vi "SLSC Parse Capabilities File.vi"(8 "error in":errorcluster, 11 "module capabilities JSON string":string) -> (0 "error out":errorcluster, 3 "SLSC EDS module":T1)   [LabVIEW 2015]
doc: "This SLSC capabilities string parser deserializes a module's JSON capabilities string as read using SLSC Read NVMEM.vi example (*.bin)) and converts it to a cluster."
uses:
  EDSjsonStructure.ctl
  enum.ctl
  property.ctl
  command.ctl
  scale.ctl
  physicalChannel.ctl
  register.ctl
  <vilib>/addons/_JKI.lib/Serialization/JSON/JKI JSON Serialization.lvlib
panel:
  out "First Region":string
  out "raw?":bool
  out "result string":string
  # "not working\nregisterMap->registers->initialValue"
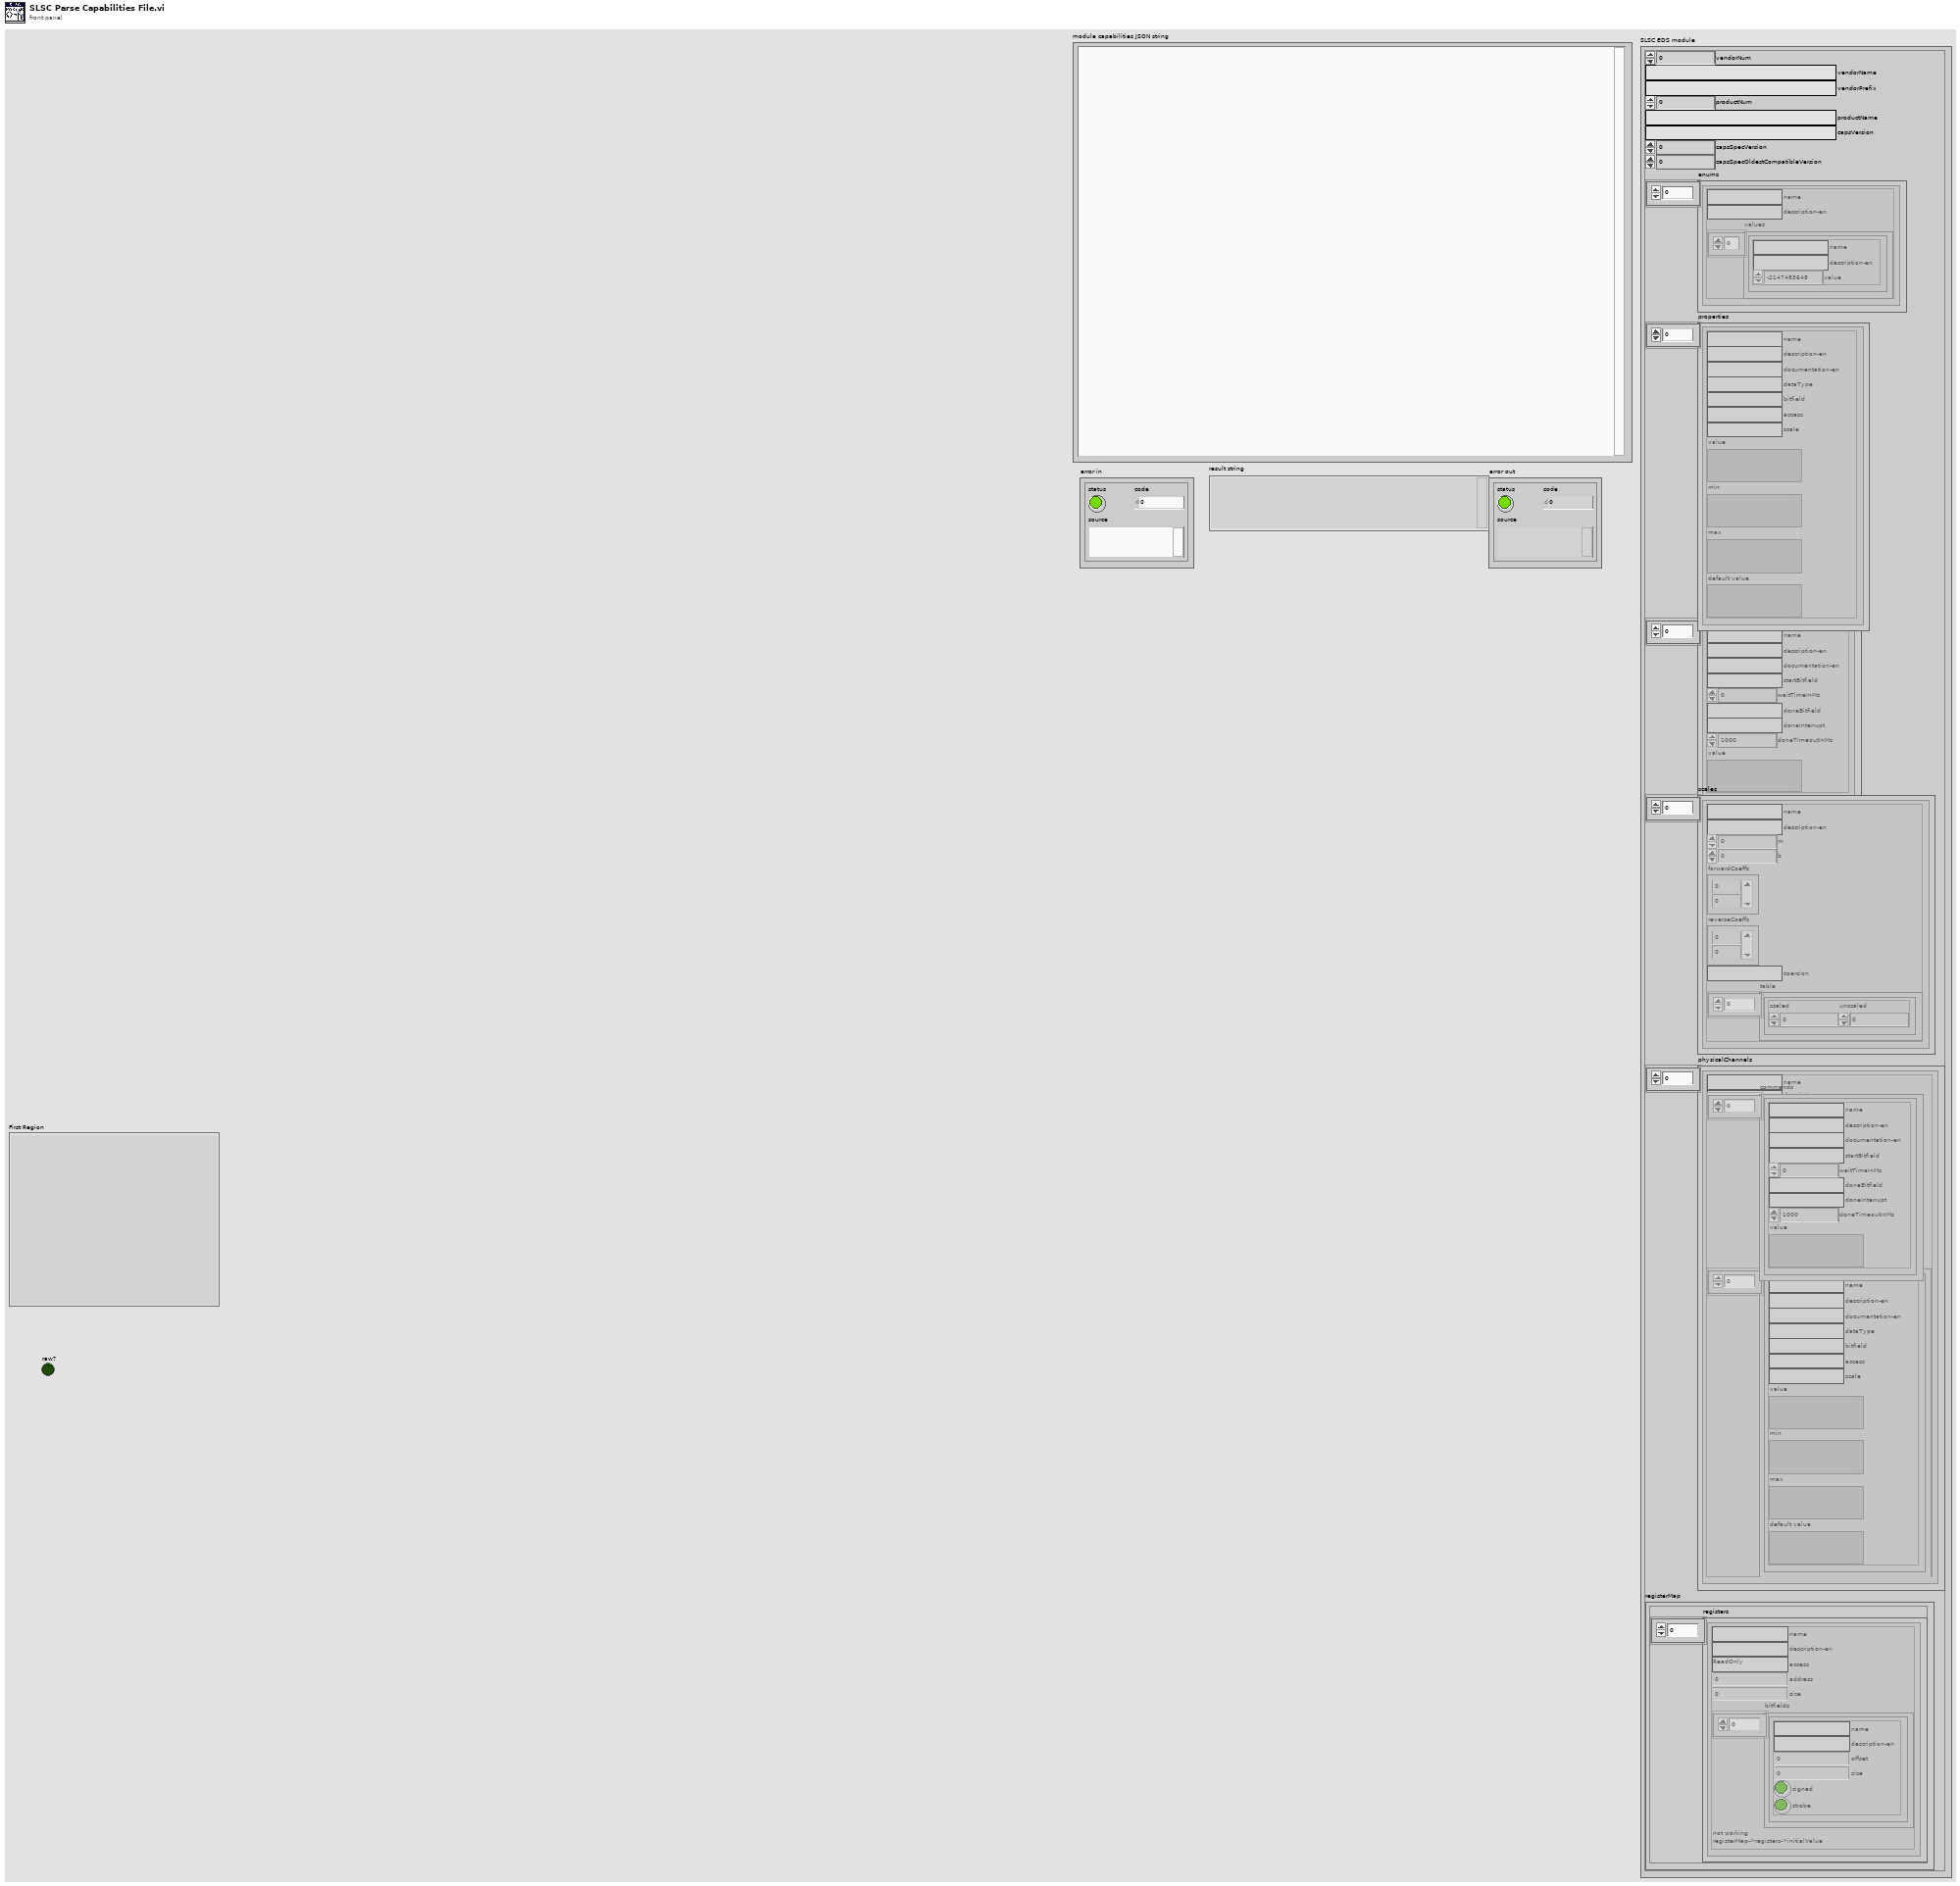
[diagram p1: front panel]
types:
  T1 = typedef "EDSjsonStructure.ctl" = cluster{"vendorNum":u32, "vendorName":string, "vendorPrefix":string, "productNum":u32, "productName":string, "capsVersion":string, "capsSpecVersion":u32, "capsSpecOldestCompatibleVersion":u32, "enums":T2[], "properties":T3[], "commands":T4[], "scales":T5[], "physicalChannels":T6[], "registerMap":cluster{"registers":T7[]}}
  T2 = typedef "enum.ctl" = cluster{"name":string, "description-en":string, "values":cluster{"name":string, "description-en":string, "value":i32}[]}
  T3 = typedef "property.ctl" = cluster{"name":string, "description-en":string, "documentation-en":string, "dataType":string, "bitfield":string, "access":string, "scale":string, "value":variant, "min":variant, "max":variant, "default value":variant}
  T4 = typedef "command.ctl" = cluster{"name":string, "description-en":string, "documentation-en":string, "startBitfield":string, "waitTimeInMs":i32, "doneBitfield":string, "doneInterrupt":string, "doneTimeoutInMs":i32, "value":variant}
  T5 = typedef "scale.ctl" = cluster{"name":string, "description-en":string, "m":dbl, "b":dbl, "forwardCoeffs":dbl[], "reverseCoeffs":dbl[], "coercion":string, "table":cluster{"scaled":dbl, "unscaled":dbl}[]}
  T6 = typedef "physicalChannel.ctl" = cluster{"name":string, "description-en":string, "commands":T4[], "properties":T3[]}
  T7 = typedef "register.ctl" = cluster{"name":string, "description-en":string, "access":string, "address":u32, "size":u32, "bitfields":cluster{"name":string, "description-en":string, "offset":u32, "size":u32, "signed":bool, "strobe":bool}[]}
  T8 = cluster{"areas":cluster{"name":string, "offsets":i32[], "size":i32}[]}
  T9 = cluster{"name":string, "offsets":i32[], "size":i32}[]
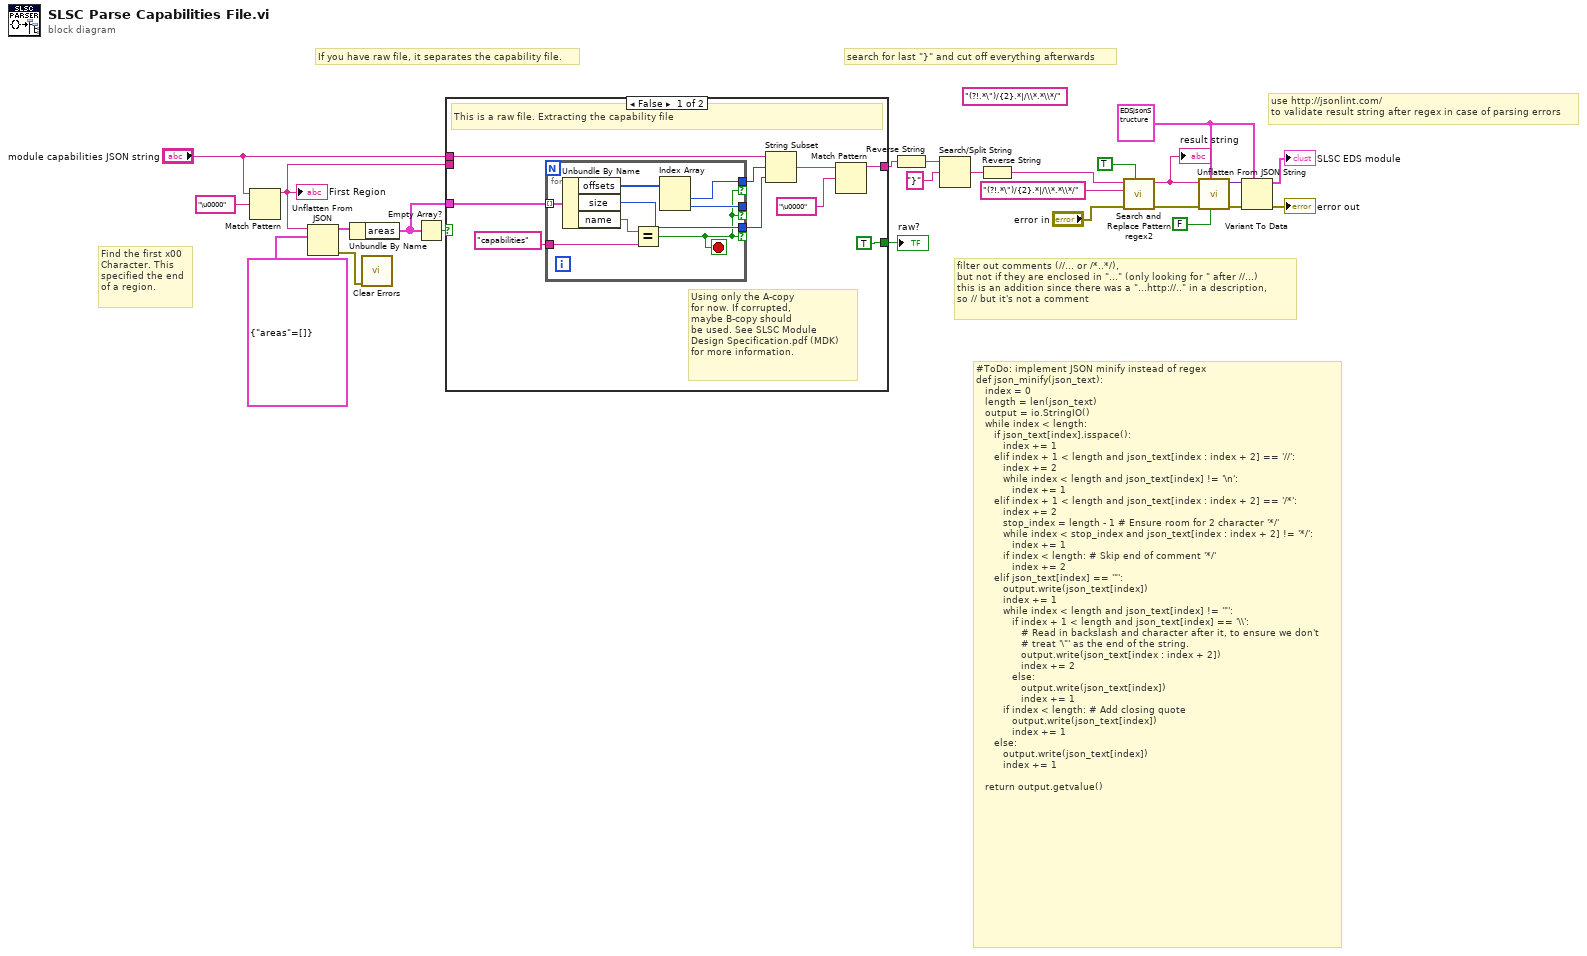
[diagram p0: block diagram]
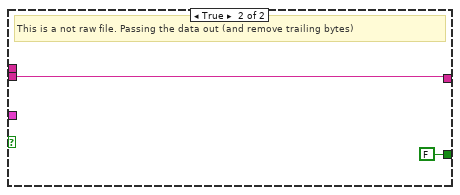
[diagram p2: hidden frame]
diagram:
  (unwired) "(?!.*\")/{2}.*|/\\*.*\\*/" ("regular expression (\"\")")
  w19 = T1 {"vendorNum"=0, "vendorName"="", "vendorPrefix"="", "productNum"=0, "productName"="", "capsVersion"="", "capsSpecVersion"=0, "capsSpecOldestCompatibleVersion"=0, "enums"=[], "properties"=[], "commands"=[], "scales"=[], "physicalChannels"=[], "registerMap"={"registers"=[]}} ("ESDmoduleOptElements")
  # "If you have raw file, it separates the capability file."
  # "Find the first x00 \nCharacter. This \nspecified the end\nof a region."
  # "#ToDo: implement JSON minify instead of regex\ndef json_minify(json_text):\n   index = 0\n   length = len(json_text)\n   output = io.StringIO()\n   while index < length:\n      if json_text[index].isspace():\n         index += 1\n      elif index + 1 < length and json_text[index : index + 2] == '//':\n         index += 2\n         while index < length and json_text[index] != '\\n':\n            index += 1\n      elif index + 1 < length and json_text[index : index + 2] == '/*':\n         index += 2\n         stop_index = length - 1 # Ensure room for 2 character '*/'\n         while index < stop_index and json_text[index : index + 2] != '*/':\n            index += 1\n         if index < length: # Skip end of comment '*/'\n            index += 2\n      elif json_text[index] == '\"':\n         output.write(json_text[index])\n         index += 1\n         while index < length and json_text[index] != '\"':\n            if index + 1 < length and json_text[index] == '\\\\':\n               # Read in backslash and character after it, to ensure we don't\n               # treat '\\\"' as the end of the string.\n               output.write(json_text[index : index + 2])\n               index += 2\n            else:\n               output.write(json_text[index])\n               index += 1\n         if index < length: # Add closing quote\n            output.write(json_text[index])\n            index += 1\n      else:\n         output.write(json_text[index])\n         index += 1\n\n   return output.getvalue()"
  # "search for last \"}\" and cut off everything afterwards"
  # "use http://jsonlint.com/\nto validate result string after regex in case of parsing errors"
  # "filter out comments (//... or /*..*/),\nbut not if they are enclosed in \"...\" (only looking for \" after //...)\nthis is an addition since there was a \"...http://..\" in a description, \nso // but it's not a comment"
  n1 = Match Pattern(string="module capabilities JSON string", regular expression="\u0000" ("search string")) -> (before substring=w6:string)  [unwired: 1 in, 3 out]
  "First Region" <- w6
  n2 = Unflatten From JSON(JSON string=w6, type and defaults=T8 {"areas"=[]}) -> (value=w10:T8, error out=w1:errorcluster)  [unwired: 5 in]
  n3 = Unbundle By Name(w10) -> ("areas"=w9:T9)
  n4 = call <vilib>:"Clear Errors.vi"("error in (no error)"=w1) -> ()  [unwired: 5 in, 2 out]
  n5 = Empty Array?(array=w9) -> (empty?=w7:bool)
  n6 = case shown="False" w7 {
    tunnel: w9 -> [w34 _]
    tunnel: "module capabilities JSON string" -> [w32 _]
    tunnel: [w27 w44] -> w3
    tunnel: w6 -> [_ w44]
    tunnel: [TRUE ("raw?") FALSE ("raw?")] -> w5
    frame False {
      # "Using only the A-copy\nfor now. If corrupted,\nmaybe B-copy should \nbe used. See SLSC Module\nDesign Specification.pdf (MDK)\nfor more information."
      # "This is a raw file. Extracting the capability file"
      n7 = for {
        tunnel: w34 -> [w42] mode=indexing
        tunnel: "capabilities" ("y") -> [w39]
        tunnel: [w38] -> w30 if=w35
        tunnel: [w37] -> w31 if=w35
        tunnel: [w36] -> _ if=w35
        stop <- w35 stop-if-true
        n8 = Unbundle By Name(w42) -> ("offsets"=w40:i32[], "size"=w38:i32, "name"=w41:string)
        n9 = Equal?(x=w41, y=w39) -> (x = y?=w35:bool)
        n10 = Index Array(array=w40) -> (element #1=w37:i32, element #2=w36:i32)  [unwired: 2 in]
      }
      n11 = String Subset(string=w32, offset (0)=w31, length (rest)=w30) -> (substring=w28:string)
      n12 = Match Pattern(string=w28, regular expression="\u0000" ("search string")) -> (before substring=w27:string)  [unwired: 1 in, 3 out]
    }
    frame True {
      # "This is a not raw file. Passing the data out (and remove trailing bytes)"
    }
  }
  "raw?" <- w5
  n13 = Reverse String(1:w3) -> (0:w15:string)
  n14 = Search/Split String(string=w15, search string/char (-)="}") -> (match + rest of string=w12:string)  [unwired: 1 in, 2 out]
  n15 = Reverse String(1:w12) -> (0:w13:string)
  n16 = call "Search and Replace Pattern regex2.vi"("replace all? (F)"=TRUE, "error in"="error in", "regular expression (\"\")"="(?!.*\")/{2}.*|/\\*.*\\*/" ("regular expression (\"\")"), "string"=w13) -> ("error out"=w17:errorcluster, "result string"=w23:string)  [unwired: 5 in, 1 out]
  "result string" <- w23
  n17 = call <vilib>:"Unflatten From JSON String.vi"("Nulls as Defaults (F)"=FALSE, "Type and Defaults"=w19, "error in (no error)"=w17, "JSON String"=w23) -> ("error out"=w22:errorcluster, "Variant"=w21:variant)  [unwired: 6 in]
  n18 = Variant To Data(error in=w22, type=w19, Variant=w21) -> (data=→"SLSC EDS module":T1, error out=→"error out":errorcluster)
